vi "Initialize.vi"(0 "instance":u8) -> (4 "subsysytem":refnum<class "Single Address Space Collection.lvclass">, 6 "AddressSpace":refnum<class "AddressSpace.lvclass">)   [LabVIEW 2017, in "ThreePhasePLL.lvlib" / "AddressSpace.lvclass"]
uses:
  AddressSpace.lvclass
  <instrlib>/_niInstr/Instruction Framework/v1/FPGA/Helper Classes/Single Address Space Collection/Single Address Space Collection.lvclass
  C:/Program Files (x86)/National Instruments/LabVIEW 2017/instr.lib/_niInstr/Instruction Framework/v1/FPGA/Interfaces/Address Space/Address Space.lvclass
  AddressSpace.lvclass/AddressSpace.ctl
  ThreePhasePLL.lvlib
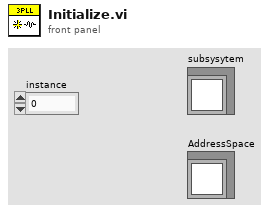
[diagram p1: front panel]
types:
  T1 = typedef "ThreePhasePLL.lvlib/registers.ctl" = cluster{"PLLGains":refnum<k21>, "PLLRange":refnum<k21>, "PLL_reset":refnum<k21>, "PLL_locked":refnum<k21>, "freqBoundaries":refnum<k21>, "expectedFreq":refnum<k21>, "lockDuration":refnum<k21>, "dT":refnum<k21>, "detectedFreq":refnum<k21>, "adjustTheta":refnum<k21>, "HarmonicFilter":refnum<k21>, "HarmonicFilterEnable":refnum<k21>}
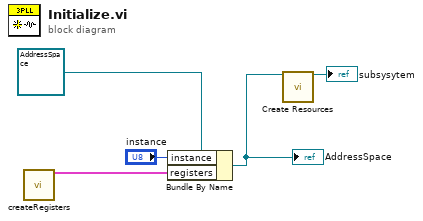
[diagram p0: block diagram]
diagram:
  n1 = call "createRegisters.vi"() -> ("registers"=w1:T1)  [unwired: 15 in]
  n2 = Bundle By Name(cluster=refnum<class "AddressSpace.lvclass"> refnum ("ThreePhasePLL.lvlib:AddressSpace.lvclass"), "instance"="instance", "registers"=w1) -> (w2:refnum<class "AddressSpace.lvclass">)
  "AddressSpace" <- w2
  n3 = call <instrlib>:"Create Resources.vi"("address space"=w2) -> ("single address space collection"=→"subsysytem":refnum<class "Single Address Space Collection.lvclass">)  [unwired: 14 in]
